vi "pico_init.vi"() -> (0 "error out 3":errorcluster, 1 "ID":i32, 2 "key":string, 3 "CmdLib Out":refnum<k24>)   [LabVIEW 2014]
uses:
  C:/Program Files/New Focus/New Focus Picomotor Application/Samples/CmdLib.dll
  Program Files/New Focus/New Focus Picomotor Application/Samples/CmdLib.dll
panel:
  out "ID List":string[](array[string])
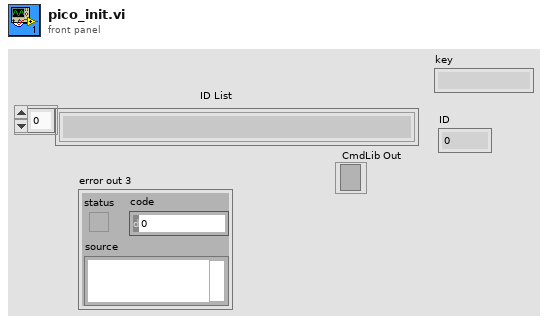
[diagram p1: front panel]
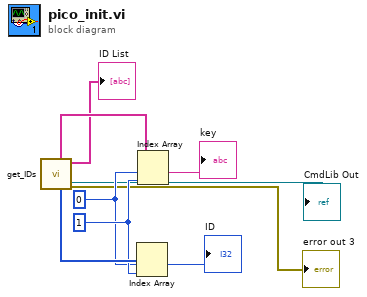
[diagram p0: block diagram]
diagram:
  w6 = 1 ("index")
  w5 = 0 ("index")
  n1 = call "get_IDs.vi"() -> ("error out 3"=→"error out 3":errorcluster, "CmdLib Out"=→"CmdLib Out":refnum<k24>, "Identification List"=→"ID List":string[], "IDs"=w7:i32[], "Device Key"=w9:string[])  [unwired: 6 in, 1 out]
  n2 = Index Array(array=w7, index #1=w5, index #2=w6) -> (element #1=→"ID":i32)  [unwired: 1 out]
  n3 = Index Array(array=w9, index #1=w5, index #2=w6) -> (element #1=→"key":string)  [unwired: 1 out]
